vi "RunLog.vi"(2 "error in":errorcluster, 3 "Message":string) -> (0 "error out":errorcluster)   [LabVIEW 2018]
panel:
  # "处理当前错误并更新当前信息"
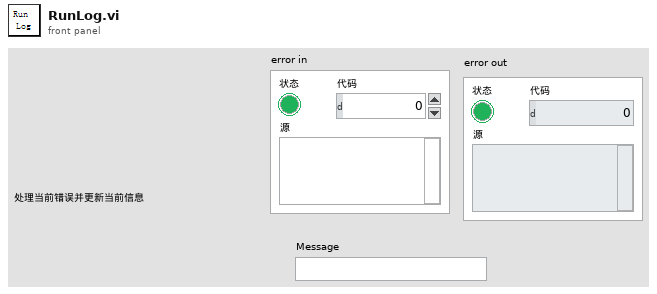
[diagram p1: front panel]
types:
  T1 = cluster{"Selected Index []":i32[], "Selected Items":string[], " 所有任务":string[], "任务布尔":bool[]}
  T2 = enum16{"光谱测量", "功率测量", "能量测量", "时间波形", "偏振测量", "近远场"}
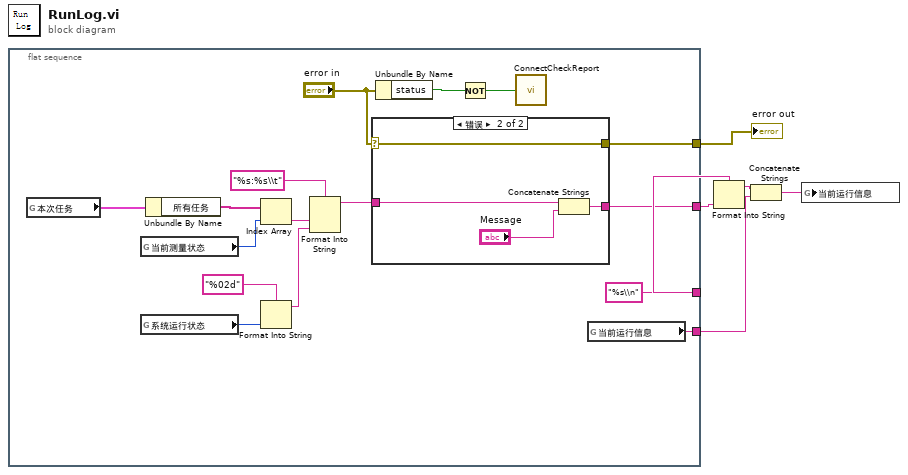
[diagram p0: block diagram]
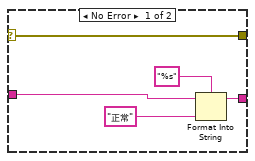
[diagram p2: hidden frame]
diagram:
  n1 = flat-sequence {
    tunnel: [w13] -> w6
    tunnel: [w12] -> w5
    tunnel: ["%s\\n" ("格式字符串")] -> w3
    tunnel: [w10] -> w2
    frame #0 {
      n2 = global read "参数.vi" "本次任务"() -> (w22:T1)
      n3 = global read "参数.vi" "当前测量状态"() -> (w17:T2)
      n4 = global read "参数.vi" "系统运行状态"() -> (w16:enum16{"通信测试", "初始化", "测量", "写入"})
      n5 = Unbundle By Name(w22) -> ("所有任务"=w21:string[])
      n6 = Index Array(array=w21, index=w17) -> (element=w19:string)
      n7 = Format Into String(format string="%02d" ("格式字符串"), w16) -> (resulting string=w14:string)  [unwired: 2 in, 1 out]
      n8 = Format Into String(format string="%s:%s\\t" ("格式字符串"), w19, w14) -> (resulting string=w18:string)  [unwired: 2 in, 1 out]
      n9 = case shown="错误" "error in" {
        selector: "error in" -> [w23 w28]
        tunnel: w18 -> [w27 w31]
        tunnel: [w24 w30] -> w10
        tunnel: [w23 w28] -> w13
        frame No Error {
          n10 = Format Into String(format string="%s" ("格式字符串"), initial string=w27, "正常" ("输入 1")) -> (resulting string=w24:string)  [unwired: 1 in, 1 out]
        }
        frame Error {
          n11 = Concatenate Strings(w31, "Message") -> (w30:string)
        }
      }
      n12 = Unbundle By Name("error in") -> ("status"=w8:bool)
      n13 = Not(x=w8) -> (.not. x?=w7:bool)
      n14 = call "ConnectCheckReport.vi"("通信状态"=w7) -> ()  [unwired: 1 in]
      n15 = global read "globalMessage.vi" "当前运行信息"() -> (w12:string)
    }
  }
  n16 = Format Into String(format string=w3, w2) -> (resulting string=w1:string)  [unwired: 2 in, 1 out]
  n17 = Concatenate Strings(w1, w5) -> (w4:string)
  n18 = global write "globalMessage.vi" "当前运行信息"(w4) -> ()
  "error out" <- w6
